vi "take step fast.vi"(7 "blocking?":bool=TRUE, 8 "error in":errorcluster, 11 "actuator in":T1={"Actuator COM"="COM14", "Actuator type"=enum."Scientifica"}) -> (0 "error out":errorcluster, 3 "actuator out":T1={"Actuator COM"="COM14", "Actuator type"=enum."Scientifica"})   [LabVIEW 2015]
uses:
  pipette cleaning/pressure box/cleaning_soft/controls/scientifica_commands.ctl
  pipette cleaning/pressure box/cleaning_soft/controls/actuator_type.ctl
  pipette cleaning/pressure box/cleaning_soft/controls/actuator_cluster.ctl
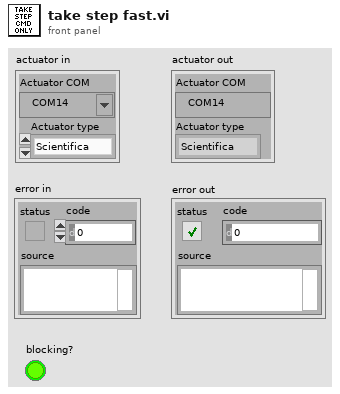
[diagram p1: front panel]
types:
  T1 = typedef "actuator_cluster.ctl" = cluster{"Actuator COM":refnum<visa-resource-name>, "Actuator type":T2}
  T2 = typedef "actuator_type.ctl" = enum16{"Scientifica", "Sutter", "Demo", "Off"}
  T3 = typedef "scientifica_commands.ctl" = enum16{"ANGLE", "INSET", "FIRST", "ZERO", "Pz", "P", "absz", "ACC", "TOP", "STOP", "rel", "relz", "abs", "IN", "vj", "APROACH", "OBJS", "OBJU", "OUT", "OBJ", "OBJL", "SET", "OBJD", "STEP", "SETSTEP", "S", "UUX", "UUY", "UUZ"}
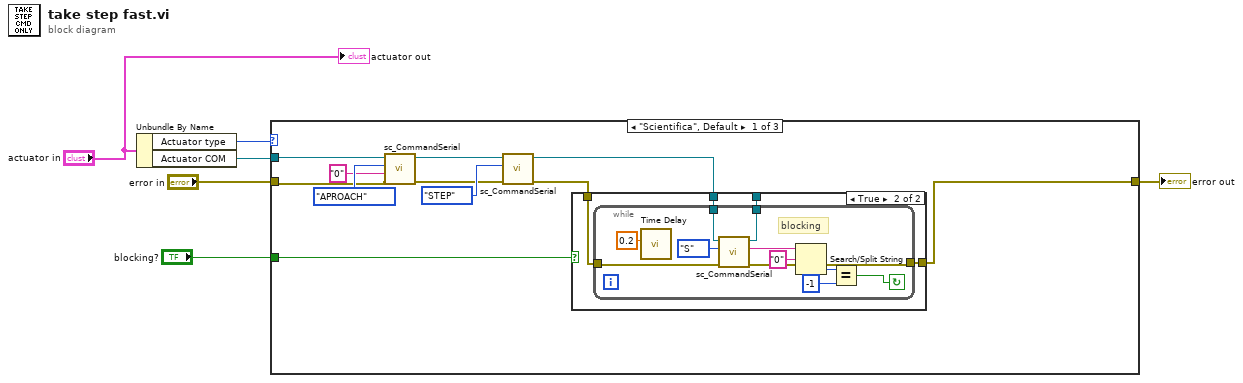
[diagram p0: block diagram]
diagram:
  n1 = Unbundle By Name("actuator in") -> ("Actuator type"=w5:T2, "Actuator COM"=w4:refnum<visa-resource-name>)
  n2 = case shown="\"Scientifica\", Default" w5 {
    tunnel: w4 -> [w10 _ _]
    tunnel: "error in" -> [w9 w35 w36]
    tunnel: [w13 w35 w36] -> w2
    tunnel: "blocking?" -> [w16 _ _]
    frame "Scientifica", Default {
      n3 = call "sc_CommandSerial.vi"("error in (no error)"=w9, "argument"="0", "Scientifica commands"=scientifica_commands."APROACH", "VISA handle"=w10) -> ("error out"=w8:errorcluster, "Dup. VISA handle"=w7:refnum<visa-resource-name>)  [unwired: 4 in, 2 out]
      n4 = call "sc_CommandSerial.vi"("error in (no error)"=w8, "Scientifica commands"=scientifica_commands."STEP", "VISA handle"=w7) -> ("error out"=w15:errorcluster, "Dup. VISA handle"=w14:refnum<visa-resource-name>)  [unwired: 5 in, 2 out]
      n5 = case shown="True" w16 {
        tunnel: w15 -> [w19 w23]
        tunnel: [w19 w22] -> w13
        tunnel: w14 -> [w18 w21]
        tunnel: [w18 w20] -> _
        frame False {
        }
        frame True {
          n6 = while {
            tunnel: w23 -> [w33]
            tunnel: [w27] -> w22
            tunnel: w21 -> [w25]
            tunnel: [w24] -> w20
            stop <- w28 continue-if-true
            # "blocking"
            n7 = call "Time Delay"("Delay Time (s)"=0.2) -> ()  [unwired: 10 in, 1 out]
            n8 = call "sc_CommandSerial.vi"("error in (no error)"=w33, "Scientifica commands"=scientifica_commands."S", "VISA handle"=w25) -> ("error out"=w27:errorcluster, "Response"=w31:string, "Dup. VISA handle"=w24:refnum<visa-resource-name>)  [unwired: 5 in, 1 out]
            n9 = Search/Split String(string=w31, search string/char (-)="0") -> (offset of match=w30:i32)  [unwired: 1 in, 2 out]
            n10 = Equal?(x=w30, y=-1) -> (x = y?=w28:bool)
          }
        }
      }
    }
    frame "Sutter" {
    }
    frame "Demo" {
    }
  }
  "error out" <- w2
  "actuator out" <- "actuator in"
